vi "BinH to BinW.vi"() -> ()   [LabVIEW 2015]
panel:
  in  "Time base":dbl=2.5e-07 format="%.4e"
  in  "Delay, points":i32=-16000
  out "new file path (Not A Path if cancelled)":path
  out "error out":errorcluster
  in  "error in (no error)":errorcluster
  in  "file path (dialog if empty)":path
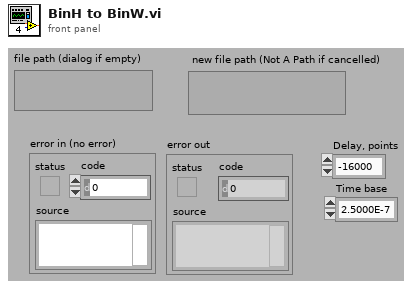
[diagram p1: front panel]
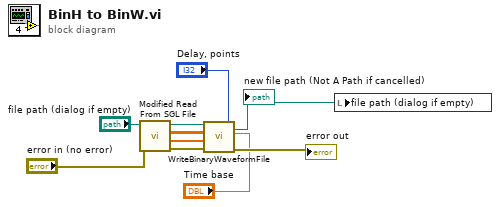
[diagram p0: block diagram]
diagram:
  n1 = call "Modified Read From SGL File.vi"("error in (no error)"="error in (no error)", "file path (dialog if empty)"="file path (dialog if empty)") -> ("error out"=w4:errorcluster, "1D array"=w7:sgl[], "2D array"=w8:sgl[][], "new file path (Not A Path if cancelled)"=w9:path)  [unwired: 4 in, 2 out]
  n2 = call "WriteBinaryWaveformFile.vi"("Time base"="Time base", "Delay, points"="Delay, points", "error in (no error)"=w4, "1D array"=w7, "2D array"=w8, "file path (dialog if empty)"=w9) -> ("error out"=→"error out":errorcluster, "new file path (Not A Path if cancelled)"=w6:path)  [unwired: 4 in]
  "new file path (Not A Path if cancelled)" <- w6
  n3 = local write "file path (dialog if empty)"(w6) -> ()
